vi "Move Enum.vi"(6 "position":T1={"Left"=-1000, "Top"=-1000}, 7 "move?":bool, 8 "error in":errorcluster, 11 "enum ref":refnum<vi>) -> (0 "error out":errorcluster)   [LabVIEW 2013, in "Table Manager.lvlib"]
uses:
  Table API/Table Manager.lvlib
  <vilib>/Utility/miscctls.llb/LVPositionTypeDef.ctl
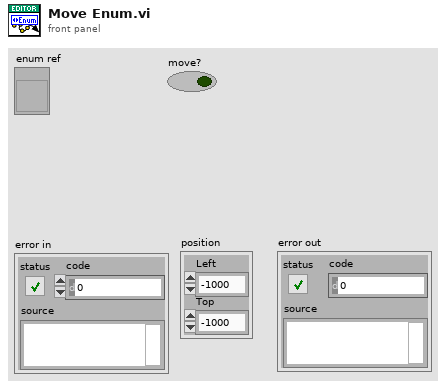
[diagram p1: front panel]
types:
  T1 = typedef "LVPositionTypeDef.ctl" = cluster{"Left":i32, "Top":i32}
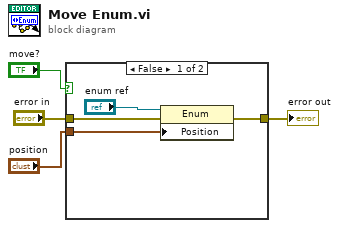
[diagram p0: block diagram]
diagram:
  n1 = case shown="False" "move?" {
    tunnel: "error in" -> [w8 w9]
    tunnel: [w6 w9] -> w4
    tunnel: "position" -> [w5 _]
    frame False {
      n2 = property on="Property Node" class="Enum"(reference="enum ref", error in=w8, "Position"=w5) -> (error out=w6:errorcluster)  [unwired: 1 out]
    }
    frame True {
    }
  }
  "error out" <- w4
